vi "Message Available.vi"(8 "error in (no error)":errorcluster, 10 "delay":u16(ring) items=["none", "error check", "multiline read", "infinite"], 11 "VISA resource name":refnum<visa-resource-name>) -> (0 "error out":errorcluster, 2 "message available":bool, 3 "VISA resource name out":refnum<visa-resource-name>)   [LabVIEW 2025, in "Andeen-Hagerling 2700A.lvlib"]
doc: "Wait for a variable delay and return a boolean to indicate if a message is available from the bridge."
uses:
  Andeen-Hagerling 2700A.lvlib
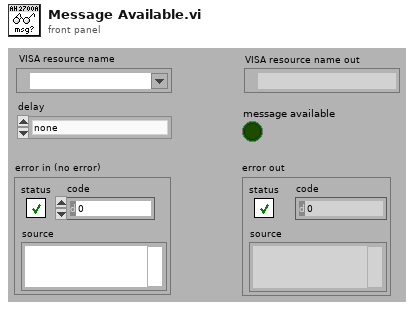
[diagram p1: front panel]
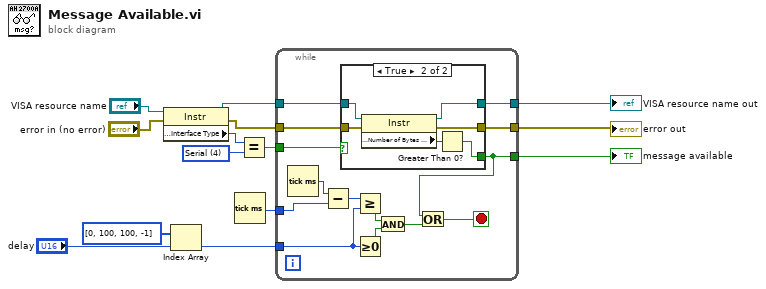
[diagram p0: block diagram]
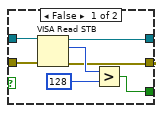
[diagram p2: hidden frame]
diagram:
  w14 = u16 4 items=["GPIB"=1, "VXI"=2, "GPIB-VXI"=3, "Serial"=4, "PXI"=5, "TCPIP"=6, "USB"=7] ("Interface Information:Interface Type")
  n1 = property class="Instr"(reference="VISA resource name", error in="error in (no error)") -> (reference out=w9:refnum<visa-resource-name>, error out=w8:errorcluster, "Interface Information:Interface Type"=w13:u16)
  n2 = Index Array(array=i16[] [0, 100, 100, -1], index="delay") -> (element=w2:i16)
  n3 = Tick Count (ms)() -> (millisecond timer value=w3:u32)
  n4 = Equal?(x=w13, y=w14) -> (x = y?=w10:bool)
  n5 = while {
    tunnel: w10 -> [w28]
    tunnel: w9 -> [w27]
    tunnel: w8 -> [w26]
    tunnel: [w25] -> w7
    tunnel: [w24] -> w6
    tunnel: [w16] -> w5
    tunnel: w3 -> [w22]
    tunnel: w2 -> [w20]
    stop <- w15 stop-if-true
    n6 = Tick Count (ms)() -> (millisecond timer value=w23:u32)
    n7 = Subtract(x=w23, y=w22) -> (x-y=w21:u32)
    n8 = case shown="True" w28 {
      tunnel: w27 -> [w33 w40]
      tunnel: w26 -> [w32 w39]
      tunnel: [w31 w38] -> w25
      tunnel: [w30 w37] -> w24
      tunnel: [w29 w36] -> w16
      frame False {
        n9 = VISA Read STB(8:w32, 11:w33) -> (0:w30:errorcluster, 2:w35:u16, 3:w31:refnum<visa-resource-name>)
        n10 = Greater?(x=w35, y=u16 128) -> (0:w29:bool)
      }
      frame True {
        n11 = property class="Instr"(reference=w40, error in=w39) -> (reference out=w38:refnum<visa-resource-name>, error out=w37:errorcluster, "Serial Settings:Number of Bytes at Serial Port"=w41:u32)
        n12 = Greater Than 0?(x=w41) -> (x > 0?=w36:bool)
      }
    }
    n13 = Greater Or Equal?(x=w21, y=w20) -> (x >= y?=w18:bool)
    n14 = Greater Or Equal To 0?(x=w20) -> (x >= 0?=w19:bool)
    n15 = And(x=w18, y=w19) -> (x .and. y?=w17:bool)
    n16 = Or(x=w16, y=w17) -> (x .or. y?=w15:bool)
  }
  "error out" <- w6
  "VISA resource name out" <- w7
  "message available" <- w5
